vi "Test Insert Tables in not existing Sheet.vi"(11 "Test Case In":refnum<class "Test Open Xml.lvclass">) -> (0 "error out":errorcluster, 3 "Test Case Out":refnum<class "Test Open Xml.lvclass">)   [LabVIEW 2020, in "Test Open Xml.lvclass"]
uses:
  Test Open Xml.lvclass
  C:/Program Files/National Instruments/LabVIEW 2025/vi.lib/Astemes/LUnit/Test Case.lvclass
  <vilib>/Astemes/LUnit/Test Case.lvclass/Test Case.ctl
  0a0d70f3-36fe-46ba-8b3e-e6c07e708d9f.vi
  <vilib>/Astemes/LUnit/Core/LUnit Test Case/Private/Append Pass Result.vi
  <vilib>/Astemes/LUnit/Core/LUnit Test Case/Private/Append Fail Result.vi
  0a0d70f3-36fe-46ba-8b3e-e6c07e708d9f.vi/9c5d11cd-9439-4240-a1ee-d9baace9c924.vi
  <vilib>/Astemes/LUnit/Core/LUnit Test Case/Private/Run In UI.vi
  <vilib>/Utility/error.llb/Clear Errors.vi
  Source/Open Xml.lvlib
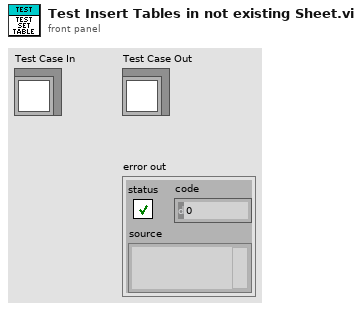
[diagram p1: front panel]
types:
  T1 = cluster{"Sheet Name":string, "Name":string, "Display Name":string, "Range or Cell Address":string}
  T2 = cluster{"Sheet Name":string, "Name":string, "Display Name":string, "Range":string}
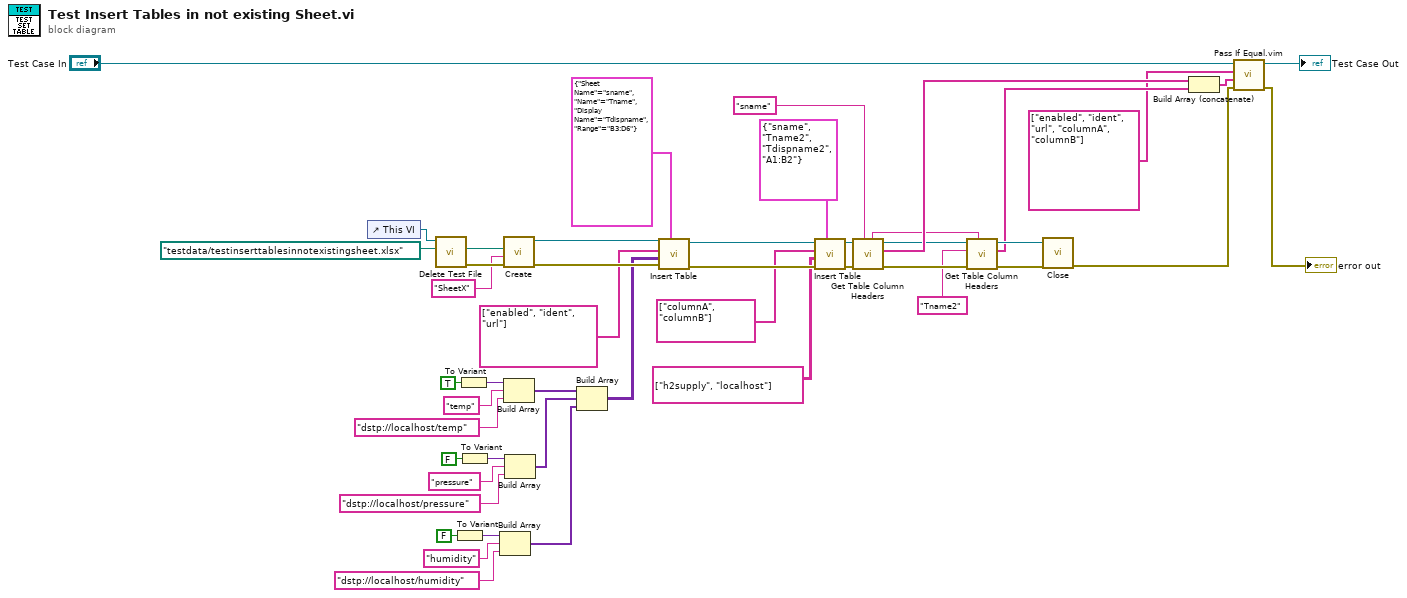
[diagram p0: block diagram]
diagram:
  n1 = control-ref of="This VI"() -> (w37:refnum<vi>)
  n2 = call "Delete Test File.vi"("name or relative path"=path "testdata/testinserttablesinnotexistingsheet.xlsx", "VI in"=w37) -> ("error out"=w38:errorcluster, "deleted path"=w39:path)  [unwired: 8 in]
  n3 = To Variant(anything=FALSE) -> (Variant=w9:variant)
  n4 = To Variant(anything=TRUE) -> (Variant=w18:variant)
  n5 = To Variant(anything=FALSE) -> (Variant=w12:variant)
  n6 = Build Array(w9, "humidity", "dstp://localhost/humidity") -> (w5:variant[])
  n7 = call "Create.vi"("error in"=w38, "SheetName"="SheetX", "Path"=w39) -> ("error out"=w34:errorcluster, "SpreadsheetDoc"=w35:refnum<k24>)  [unwired: 7 in]
  n8 = Build Array(w18, "temp", "dstp://localhost/temp") -> (w15:variant[])
  n9 = Build Array(w12, "pressure", "dstp://localhost/pressure") -> (w6:variant[])
  n10 = Build Array(w15, w6, w5) -> (w4:variant[][])
  n11 = call "Insert Table.vi"("Location"=T2 {"Sheet Name"="sname", "Name"="Tname", "Display Name"="Tdispname", "Range"="B3:D6"}, "error in"=w34, "Cell Values"=w4, "Header Names"=string[] ["enabled", "ident", "url"], "SpreadsheetDoc in"=w35) -> ("error out"=w41:errorcluster, "SpreadsheetDoc out"=w30:refnum<k24>)  [unwired: 5 in]
  n12 = call "Insert Table.vi"("Location"=T1 {"Sheet Name"="sname", "Name"="Tname2", "Display Name"="Tdispname2", "Range or Cell Address"="A1:B2"}, "error in"=w41, "Cell Values"=string[][] [["h2supply", "localhost"]], "Header Names"=string[] ["columnA", "columnB"], "SpreadsheetDoc in"=w30) -> ("error out"=w31:errorcluster, "SpreadsheetDoc out"=w29:refnum<k24>)  [unwired: 5 in]
  n13 = call "Get Table Column Headers.vi"("Sheet Name in"="sname", "error in"=w31, "SpreadsheetDoc in"=w29) -> ("error out"=w43:errorcluster, "Headers"=w42:string[], "SpreadsheetDoc out"=w25:refnum<k24>, "Sheet Name out"=w1:string)  [unwired: 5 in]
  n14 = call "Get Table Column Headers.vi"("Sheet Name in"=w1, "error in"=w43, "Table Name"="Tname2", "SpreadsheetDoc in"=w25) -> ("error out"=w26:errorcluster, "Headers"=w22:string[], "SpreadsheetDoc out"=w24:refnum<k24>)  [unwired: 4 in, 1 out]
  n15 = call "Close.vi"("error in"=w26, "SpreadsheetDoc"=w24) -> ("error out"=w44:errorcluster)  [unwired: 9 in]
  n16 = Build Array (concatenate)(w42, w22) -> (w23:string[])
  n17 = call "Pass If Equal.vim"("error in (no error)"=w44, "Actual"=w23, "Expected"=string[] ["enabled", "ident", "url", "columnA", "columnB"] ("Headers"), "LUnit Test Case In"="Test Case In") -> ("error out"=→"error out":errorcluster, "LUnit Test Case Out"=→"Test Case Out":refnum<class "Test Open Xml.lvclass">)  [unwired: 6 in]
